vi "GetDisplayItems__slk_mt.vi"(8 "error in (no error)":errorcluster, 11 "tree view in":refnum<class "TreeView__slk_mt.lvclass">) -> (0 "error out":errorcluster, 3 "tree view out":refnum<class "TreeView__slk_mt.lvclass">)   [LabVIEW 2020, in "TreeView__slk_mt.lvclass"]
doc: "Gets display items and theirs open status."
uses:
  TreeView__slk_mt.lvclass
  TreeView__slk_mt.lvclass/TreeView__slk_mt.ctl
panel:
  # "GetDisplayItems__slk_mt.vi\nGets display items and theirs open status.\n\nNOTICE -- YOU MUST LEAVE THIS NOTICE IN PLACE.\n\nCopyright (c) 2011, LIANG LIU Shawn.Liu.cn@gmail.com\nAll rights reserved.\n\nRedistribution and use in source and binary forms, with or without modification, are permitted provided that the following conditions are met:\n-Redistributions of source code must retain the above copyright notice, this list of conditions and the following disclaimer.\n-Redistributions in binary form must reproduce the above copyright notice, this list of conditions and the following disclaimer in the documentation and/or other materials provided with the distribution.\n-Neither the name of the eLp nor the names of its contributors may be used to endorse or promote products derived from this software without specific prior written permission.\n\nTHIS SOFTWARE IS PROVIDED BY THE COPYRIGHT HOLDERS AND CONTRIBUTORS \"AS IS\" AND ANY EXPRESS OR IMPLIED WARRANTIES, INCLUDING, BUT NOT LIMITED TO, THE IMPLIED WARRANTIES OF MERCHANTABILITY AND FITNESS FOR A PARTICULAR PURPOSE ARE DISCLAIMED. IN NO EVENT SHALL THE COPYRIGHT HOLDER OR CONTRIBUTORS BE LIABLE FOR ANY DIRECT, INDIRECT, INCIDENTAL, SPECIAL, EXEMPLARY, OR CONSEQUENTIAL DAMAGES (INCLUDING, BUT NOT LIMITED TO, PROCUREMENT OF SUBSTITUTE GOODS OR SERVICES; LOSS OF USE, DATA, OR PROFITS; OR BUSINESS INTERRUPTION) HOWEVER CAUSED AND ON ANY THEORY OF LIABILITY, WHETHER IN CONTRACT, STRICT LIABILITY, OR TORT (INCLUDING NEGLIGENCE OR OTHERWISE) ARISING IN ANY WAY OUT OF THE USE OF THIS SOFTWARE, EVEN IF ADVISED OF THE POSSIBILITY OF SUCH DAMAGE."
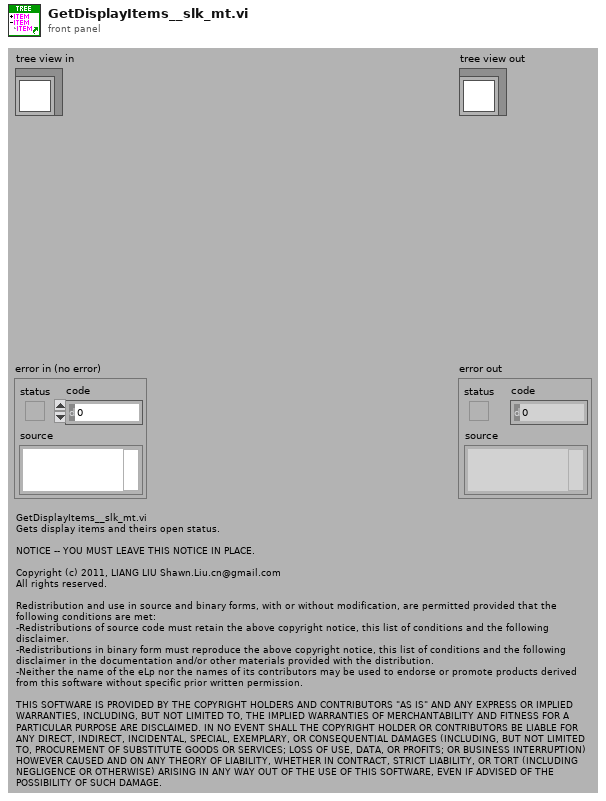
[diagram p1: front panel]
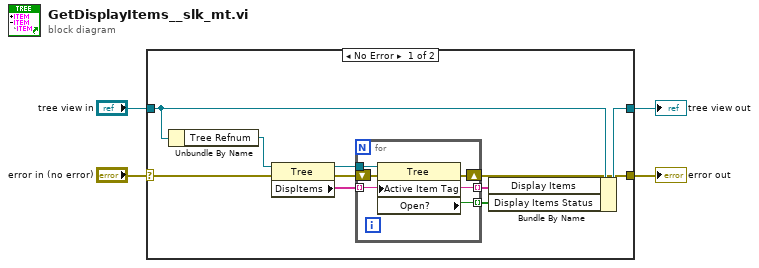
[diagram p0: block diagram]
diagram:
  n1 = case shown="No Error" "error in (no error)" {
    selector: "error in (no error)" -> [w10 w21]
    tunnel: [w5 w21] -> w3
    tunnel: [w6 w20] -> w1
    tunnel: "tree view in" -> [w7 w20]
    frame No Error {
      n2 = Unbundle By Name(w7) -> ("Tree Refnum"=w14:refnum<vi>)
      n3 = property class="Tree"(reference=w14, error in=w10) -> (reference out=w11:refnum<vi>, error out=w12:errorcluster, "DispItems"=w13:string[])
      n4 = for {
        tunnel: w13 -> [w15] mode=indexing
        shift-right: [w16] -> w5
        shift-left: w12 -> [w18]
        tunnel: w11 -> [w19]
        tunnel: [w17] -> w8 mode=indexing
        tunnel: [w15] -> w9 mode=indexing
        n5 = property class="Tree"(reference=w19, error in=w18, "Active Item Tag"=w15) -> (error out=w16:errorcluster, "Open?"=w17:bool)  [unwired: 1 out]
      }
      n6 = Bundle By Name(cluster=w7, "Display Items"=w9, "Display Items Status"=w8) -> (w6:refnum<class "TreeView__slk_mt.lvclass">)
    }
    frame Error {
    }
  }
  "error out" <- w3
  "tree view out" <- w1
